vi "Frame create.vi"(7 "Command":string, 8 "error in (no error)":errorcluster, 11 "Felica DOWN in":refnum<class "Felica DOWN.lvclass">) -> (0 "error out":errorcluster, 3 "Felica DOWN out":refnum<class "Felica DOWN.lvclass">)   [LabVIEW 2019, in "Felica DOWN.lvclass"]
uses:
  Felica DOWN.lvclass
  TypeDef/Store.ctl
  Felica DOWN.lvclass/Felica DOWN.ctl
  RFID system.lvclass
panel:
  in  "Preambul":u8[](array[numeric])=[0, 0, 0, 0, 0, 0] format="%x"
  in  "SYNC":u8[](array[numeric])=[178, 212] format="%x"
  in  "nfcid":u8[](array[numeric])=[1, 2, 3, 4, 5, 1, 2, 3, 4, 5] format="%x"
  in  "DID":u8[](array[numeric])=[20] format="%x"
  in  "CMD2":u8[](array[numeric])=[2] format="%x"
  in  "CMD1":u8[](array[numeric])=[212] format="%x"
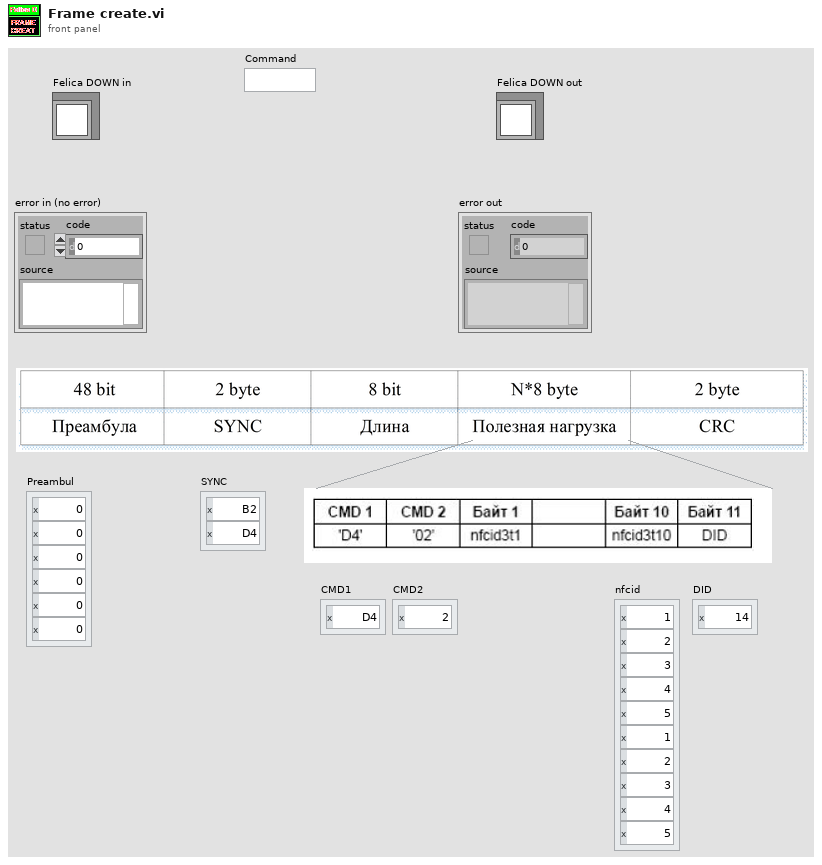
[diagram p1: front panel]
types:
  T1 = typedef "Store.ctl" = enum16{"envelope", "noise", "demSubCar", "CH_frame", "Decode", "demodulate", "in", "out", "sum", "subCarrier", "frame", "command", "encode", "modulate", "encode_UP", "modulate_up", "demod_up", "envelop_up", "sum_up", "out_up", "in_up"}
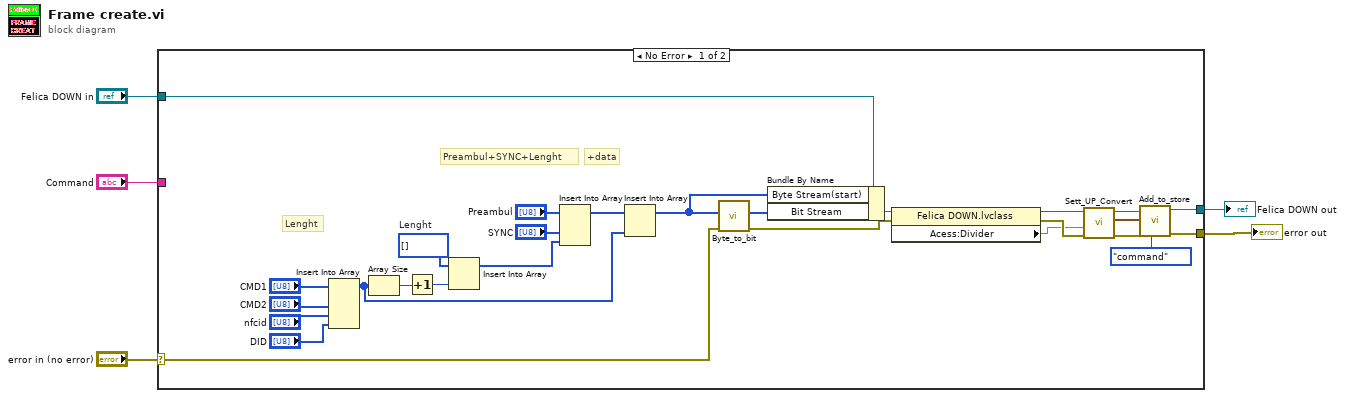
[diagram p0: block diagram]
diagram:
  n1 = case shown="No Error" "error in (no error)" {
    selector: "error in (no error)" -> [w32 w33]
    tunnel: "Felica DOWN in" -> [w26 w34]
    tunnel: [w25 w34] -> w3
    tunnel: [w24 w33] -> w2
    tunnel: "Command" -> [_ _]
    frame No Error {
      w12 = u8[] []  # Lenght
      # "+data"
      # "Preambul+SYNC+Lenght"
      # "Lenght"
      n2 = Insert Into Array(array="CMD1", new element #1="CMD2", new element #2="nfcid", new element #3="DID") -> (w23:u8[])  [unwired: 1 in]
      n3 = Array Size(array=w23) -> (size(s)=w17:i32)
      n4 = Increment(x=w17) -> (x+1=w18:i32)
      n5 = Insert Into Array(array=w12, new element=w18) -> (w21:u8[])  [unwired: 1 in]
      n6 = Insert Into Array(array="Preambul", new element #1="SYNC", new element #2=w21) -> (w22:u8[])  [unwired: 1 in]
      n7 = Insert Into Array(array=w22, new element=w23) -> (w6:u8[])  [unwired: 1 in]
      n8 = call "Byte_to_bit.vi"("Error In"=w32, "Array of byte"=w6) -> ("Error Out"=w9:errorcluster, "Arrray of bit"=w28:u8[])  [unwired: 5 in, 1 out]
      n9 = Bundle By Name(cluster=w26, "Byte Stream(start)"=w6, "Bit Stream"=w28) -> (w11:refnum<class "Felica DOWN.lvclass">)
      n10 = property class="Felica DOWN.lvclass"(reference=w11, error in=w9) -> (reference out=w10:refnum<class "Felica DOWN.lvclass">, error out=w8:errorcluster, "Acess:Divider"=w7:dbl)
      n11 = call-dynamic "Sett_UP_Convert.vi"("error in (no error)"=w8, "Divider(1)"=w7, "Felica DOWN in"=w10) -> ("error out"=w30:errorcluster, "Waveform"=w29:waveform(dbl), "Felica DOWN out"=w31:refnum<class "Felica DOWN.lvclass">)  [unwired: 6 in]
      n12 = call "Add_to_store.vi"("Store"=Store."command", "error in (no error)"=w30, "Waveform"=w29, "RFID system in"=w31) -> ("error out"=w24:errorcluster, "RFID system out"=w25:refnum<class "Felica DOWN.lvclass">)  [unwired: 6 in]
    }
    frame Error {
    }
  }
  "error out" <- w2
  "Felica DOWN out" <- w3
